vi "Post-Build Action.vi"(5 "Files Generated by Build":path[](array[path]), 6 "Top Level/Always Included VIs":path[](array[path]), 7 "Destination Path":path, 8 "error in (no error)":errorcluster, 9 "Target Name":string, 10 "Build Specification Name":string, 11 "Project Path":path) -> (0 "error out":errorcluster)   [LabVIEW 2014]
uses:
  <vilib>/Utility/config.llb/Write Key (String).vi
  <vilib>/Utility/config.llb/NI_LVConfig.lvlib
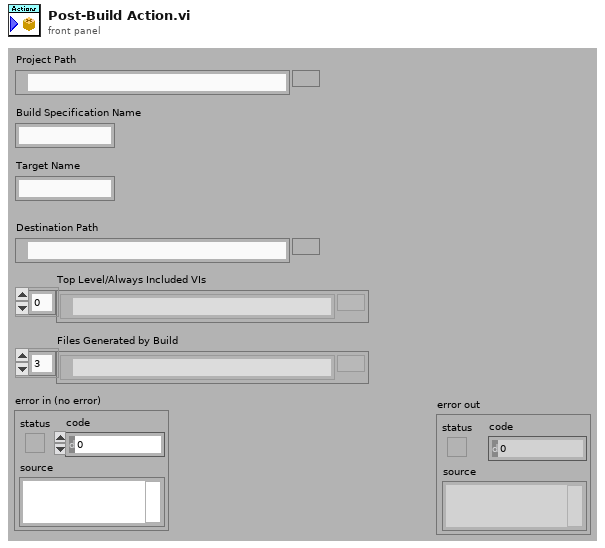
[diagram p1: front panel]
types:
  T1 = typedef "NI_LVConfig.lvlib/Config Data RefNum.ctl" = refnum<k1>
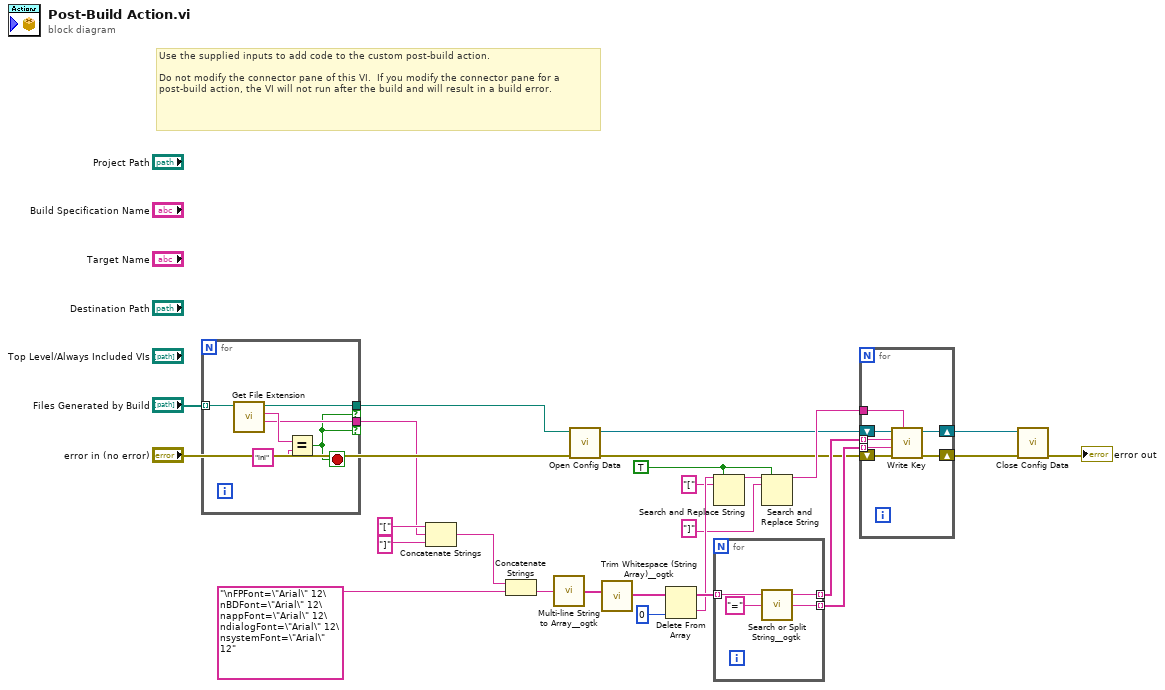
[diagram p0: block diagram]
diagram:
  w13 = TRUE ("replace all? (F)")
  # "Use the supplied inputs to add code to the custom post-build action.\n\nDo not modify the connector pane of this VI.  If you modify the connector pane for a post-build action, the VI will not run after the build and will result in a build error."
  n1 = for {
    tunnel: "Files Generated by Build" -> [w32] mode=indexing
    tunnel: [w31] -> w1 if=w27
    tunnel: [w28] -> w2 if=w27
    stop <- w27 stop-if-true
    n2 = call <vilib>:"Get File Extension.vi"("file"=w32) -> ("filename without extension"=w28:string, "lowercase file extension"=w30:string, "dup file"=w31:path)  [unwired: 7 in, 1 out]
    n3 = Equal?(x=w30, y="ini" ("string")) -> (x = y?=w27:bool)
  }
  n4 = Concatenate Strings("[" ("string"), w2, "]" ("string")) -> (w4:string)
  n5 = Concatenate Strings(w4, "\nFPFont=\"Arial\" 12\nBDFont=\"Arial\" 12\nappFont=\"Arial\" 12\ndialogFont=\"Arial\" 12\nsystemFont=\"Arial\" 12" ("String")) -> (w7:string)
  n6 = call <userlib>:"Multi-line String to Array__ogtk.vi"("string"=w7) -> ("lines"=w20:string[])
  n7 = call <vilib>:"Open Config Data.vi"("error in (no error)"="error in (no error)", "configuration file path"=w1) -> ("error out"=w9:errorcluster, "refnum"=w12:T1)  [unwired: 7 in, 1 out]
  n8 = call <userlib>:"Trim Whitespace (String Array)__ogtk.vi"("String in"=w20) -> ("String out"=w21:string[])  [unwired: 6 in]
  n9 = Delete From Array(array=w21, index=0) -> (deleted portion=w18:string, array with subset deleted=w23:string[])  [unwired: 1 in]
  n10 = Search and Replace String(replace all?=w13, input string=w18, search string="[") -> (result string=w16:string)  [unwired: 5 in, 3 out]
  n11 = for {
    tunnel: w23 -> [w36] mode=indexing
    tunnel: [w34] -> w24 mode=indexing
    tunnel: [w33] -> w25 mode=indexing
    n12 = call <userlib>:"Search or Split String__ogtk.vi"("search string/char (-)"="=", "string"=w36) -> ("substring after match"=w33:string, "substring before match"=w34:string)  [unwired: 1 in, 1 out]
  }
  n13 = Search and Replace String(replace all?=w13, input string=w16, search string="]") -> (result string=w17:string)  [unwired: 5 in, 3 out]
  n14 = for {
    tunnel: w17 -> [w39]
    shift-right: [w41] -> w10
    shift-left: w12 -> [w43]
    shift-right: [w40] -> w8
    shift-left: w9 -> [w42]
    tunnel: w24 -> [w38] mode=indexing
    tunnel: w25 -> [w37] mode=indexing
    n15 = call-poly <vilib>:"Write Key.vi"("section"=w39, "error in (no error)"=w42, "value"=w37, "key"=w38, "refnum"=w43) -> ("error out"=w40:errorcluster, "refnum out"=w41:T1)  [unwired: 4 in, 1 out]
  }
  n16 = call <vilib>:"Close Config Data.vi"("error in (no error)"=w8, "refnum"=w10) -> ("error out"=→"error out":errorcluster)  [unwired: 8 in, 1 out]
